vi "Calculate Flattened Indexes.vi"(4 "Q2 Q3 modifier (unreleased)":refnum<class "1D Array f32.lvclass">, 6 "Angle":refnum<class "1D Array f32.lvclass">, 7 "Image Size":sgl, 8 "error in (no error)":errorcluster, 9 "Relative X (unreleased)":refnum<class "1D Array f32.lvclass">, 10 "Relative Y (unreleased)":refnum<class "1D Array f32.lvclass">, 11 "Range In (unreleased)":refnum<class "2D Array f32.lvclass">) -> (0 "error out":errorcluster, 3 "Range Out":refnum<class "2D Array f32.lvclass">)   [LabVIEW 2020, in "G2CPU Line Profile.lvlib"]
uses:
  G2CPU Line Profile.lvlib
  <vilib>/Natan Biesmans/G2CPU GPU and CPU HPC Toolkit/G2CPU Libraries/Arrays/2DArray/f32/2D Array f32.lvclass
  C:/Program Files/National Instruments/LabVIEW 2025/vi.lib/Natan Biesmans/G2CPU GPU and CPU HPC Toolkit/G2CPU Libraries/Arrays/Array/Array Prototype.lvclass
  <vilib>/Natan Biesmans/G2CPU GPU and CPU HPC Toolkit/G2CPU Libraries/Arrays/1DArray/f32/1D Array f32.lvclass
  <vilib>/Natan Biesmans/G2CPU GPU and CPU HPC Toolkit/G2CPU Libraries/Arrays/Array/Array Prototype.lvclass/Array Prototype.ctl
  d14302c9-1abf-46cd-b8e1-cfd88139205b.vi
  3f418511-01e8-4418-a7b9-049296d044c6.vi
  6ff3651a-7429-4d59-9dc9-6d2307288a37.vi
  9237495b-07c2-4526-b901-02e97fb6c373.vi
  5aff2ad7-f89e-4eb8-8bcb-749f2898e5ad.vi
  8b20bb11-a6a9-4062-83c0-ddef68e428b2.vi
  <vilib>/Natan Biesmans/G2CPU GPU and CPU HPC Toolkit/G2CPU Libraries/Arrays/Array/G2CPU Get Array Pointer.vi
  d14302c9-1abf-46cd-b8e1-cfd88139205b.vi/6197f869-f6d4-49b3-9b2c-cc979b422c2e.vi
  d14302c9-1abf-46cd-b8e1-cfd88139205b.vi/a7e86dbb-b4c0-485c-89c5-522e60ee265c.vi
  3f418511-01e8-4418-a7b9-049296d044c6.vi/5793b77b-c002-4ebf-9075-685617c95341.vi
  3f418511-01e8-4418-a7b9-049296d044c6.vi/2ed3ef86-c00d-4d71-b84c-20267a6dfcf9.vi
  6ff3651a-7429-4d59-9dc9-6d2307288a37.vi/5793b77b-c002-4ebf-9075-685617c95341.vi
  6ff3651a-7429-4d59-9dc9-6d2307288a37.vi/2ed3ef86-c00d-4d71-b84c-20267a6dfcf9.vi
  9237495b-07c2-4526-b901-02e97fb6c373.vi/6197f869-f6d4-49b3-9b2c-cc979b422c2e.vi
  9237495b-07c2-4526-b901-02e97fb6c373.vi/a7e86dbb-b4c0-485c-89c5-522e60ee265c.vi
  5aff2ad7-f89e-4eb8-8bcb-749f2898e5ad.vi/6197f869-f6d4-49b3-9b2c-cc979b422c2e.vi
  5aff2ad7-f89e-4eb8-8bcb-749f2898e5ad.vi/a7e86dbb-b4c0-485c-89c5-522e60ee265c.vi
  8b20bb11-a6a9-4062-83c0-ddef68e428b2.vi/5793b77b-c002-4ebf-9075-685617c95341.vi
  8b20bb11-a6a9-4062-83c0-ddef68e428b2.vi/2ed3ef86-c00d-4d71-b84c-20267a6dfcf9.vi
  d14302c9-1abf-46cd-b8e1-cfd88139205b.vi/6197f869-f6d4-49b3-9b2c-cc979b422c2e.vi/3e802c67-fb96-46a3-ae13-4994a8508b4f.vi
  d14302c9-1abf-46cd-b8e1-cfd88139205b.vi/6197f869-f6d4-49b3-9b2c-cc979b422c2e.vi/5a50fc67-79e7-4972-80c2-92243cd53dd4.vi
  d14302c9-1abf-46cd-b8e1-cfd88139205b.vi/6197f869-f6d4-49b3-9b2c-cc979b422c2e.vi/1c928fc9-710a-40e7-8c4f-08a1069452ae.vi
  d14302c9-1abf-46cd-b8e1-cfd88139205b.vi/a7e86dbb-b4c0-485c-89c5-522e60ee265c.vi/730f6c57-5c0b-4ee9-b61e-75067b25222b.vi
  d14302c9-1abf-46cd-b8e1-cfd88139205b.vi/a7e86dbb-b4c0-485c-89c5-522e60ee265c.vi/096b8799-7810-404e-baca-ba9279cec4bd.vi
  d14302c9-1abf-46cd-b8e1-cfd88139205b.vi/a7e86dbb-b4c0-485c-89c5-522e60ee265c.vi/0f1a5a47-bcc5-4796-ac31-8dfcfbc0d7d1.vi
  d14302c9-1abf-46cd-b8e1-cfd88139205b.vi/a7e86dbb-b4c0-485c-89c5-522e60ee265c.vi/89f12e17-3330-4b72-ad8f-8dd636660732.vi
  3f418511-01e8-4418-a7b9-049296d044c6.vi/5793b77b-c002-4ebf-9075-685617c95341.vi/3e802c67-fb96-46a3-ae13-4994a8508b4f.vi
  3f418511-01e8-4418-a7b9-049296d044c6.vi/5793b77b-c002-4ebf-9075-685617c95341.vi/5a50fc67-79e7-4972-80c2-92243cd53dd4.vi
  3f418511-01e8-4418-a7b9-049296d044c6.vi/2ed3ef86-c00d-4d71-b84c-20267a6dfcf9.vi/730f6c57-5c0b-4ee9-b61e-75067b25222b.vi
  3f418511-01e8-4418-a7b9-049296d044c6.vi/2ed3ef86-c00d-4d71-b84c-20267a6dfcf9.vi/096b8799-7810-404e-baca-ba9279cec4bd.vi
  3f418511-01e8-4418-a7b9-049296d044c6.vi/2ed3ef86-c00d-4d71-b84c-20267a6dfcf9.vi/0f1a5a47-bcc5-4796-ac31-8dfcfbc0d7d1.vi
  3f418511-01e8-4418-a7b9-049296d044c6.vi/2ed3ef86-c00d-4d71-b84c-20267a6dfcf9.vi/89f12e17-3330-4b72-ad8f-8dd636660732.vi
  6ff3651a-7429-4d59-9dc9-6d2307288a37.vi/5793b77b-c002-4ebf-9075-685617c95341.vi/3e802c67-fb96-46a3-ae13-4994a8508b4f.vi
  6ff3651a-7429-4d59-9dc9-6d2307288a37.vi/5793b77b-c002-4ebf-9075-685617c95341.vi/5a50fc67-79e7-4972-80c2-92243cd53dd4.vi
  6ff3651a-7429-4d59-9dc9-6d2307288a37.vi/5793b77b-c002-4ebf-9075-685617c95341.vi/1c928fc9-710a-40e7-8c4f-08a1069452ae.vi
  6ff3651a-7429-4d59-9dc9-6d2307288a37.vi/2ed3ef86-c00d-4d71-b84c-20267a6dfcf9.vi/730f6c57-5c0b-4ee9-b61e-75067b25222b.vi
  6ff3651a-7429-4d59-9dc9-6d2307288a37.vi/2ed3ef86-c00d-4d71-b84c-20267a6dfcf9.vi/096b8799-7810-404e-baca-ba9279cec4bd.vi
  6ff3651a-7429-4d59-9dc9-6d2307288a37.vi/2ed3ef86-c00d-4d71-b84c-20267a6dfcf9.vi/0f1a5a47-bcc5-4796-ac31-8dfcfbc0d7d1.vi
  6ff3651a-7429-4d59-9dc9-6d2307288a37.vi/2ed3ef86-c00d-4d71-b84c-20267a6dfcf9.vi/89f12e17-3330-4b72-ad8f-8dd636660732.vi
  9237495b-07c2-4526-b901-02e97fb6c373.vi/6197f869-f6d4-49b3-9b2c-cc979b422c2e.vi/3e802c67-fb96-46a3-ae13-4994a8508b4f.vi
  9237495b-07c2-4526-b901-02e97fb6c373.vi/6197f869-f6d4-49b3-9b2c-cc979b422c2e.vi/5a50fc67-79e7-4972-80c2-92243cd53dd4.vi
  9237495b-07c2-4526-b901-02e97fb6c373.vi/a7e86dbb-b4c0-485c-89c5-522e60ee265c.vi/730f6c57-5c0b-4ee9-b61e-75067b25222b.vi
  9237495b-07c2-4526-b901-02e97fb6c373.vi/a7e86dbb-b4c0-485c-89c5-522e60ee265c.vi/096b8799-7810-404e-baca-ba9279cec4bd.vi
  9237495b-07c2-4526-b901-02e97fb6c373.vi/a7e86dbb-b4c0-485c-89c5-522e60ee265c.vi/0f1a5a47-bcc5-4796-ac31-8dfcfbc0d7d1.vi
  9237495b-07c2-4526-b901-02e97fb6c373.vi/a7e86dbb-b4c0-485c-89c5-522e60ee265c.vi/89f12e17-3330-4b72-ad8f-8dd636660732.vi
  5aff2ad7-f89e-4eb8-8bcb-749f2898e5ad.vi/6197f869-f6d4-49b3-9b2c-cc979b422c2e.vi/3e802c67-fb96-46a3-ae13-4994a8508b4f.vi
  5aff2ad7-f89e-4eb8-8bcb-749f2898e5ad.vi/6197f869-f6d4-49b3-9b2c-cc979b422c2e.vi/5a50fc67-79e7-4972-80c2-92243cd53dd4.vi
  5aff2ad7-f89e-4eb8-8bcb-749f2898e5ad.vi/a7e86dbb-b4c0-485c-89c5-522e60ee265c.vi/730f6c57-5c0b-4ee9-b61e-75067b25222b.vi
  5aff2ad7-f89e-4eb8-8bcb-749f2898e5ad.vi/a7e86dbb-b4c0-485c-89c5-522e60ee265c.vi/096b8799-7810-404e-baca-ba9279cec4bd.vi
  5aff2ad7-f89e-4eb8-8bcb-749f2898e5ad.vi/a7e86dbb-b4c0-485c-89c5-522e60ee265c.vi/0f1a5a47-bcc5-4796-ac31-8dfcfbc0d7d1.vi
  5aff2ad7-f89e-4eb8-8bcb-749f2898e5ad.vi/a7e86dbb-b4c0-485c-89c5-522e60ee265c.vi/89f12e17-3330-4b72-ad8f-8dd636660732.vi
  8b20bb11-a6a9-4062-83c0-ddef68e428b2.vi/5793b77b-c002-4ebf-9075-685617c95341.vi/3e802c67-fb96-46a3-ae13-4994a8508b4f.vi
  8b20bb11-a6a9-4062-83c0-ddef68e428b2.vi/5793b77b-c002-4ebf-9075-685617c95341.vi/5a50fc67-79e7-4972-80c2-92243cd53dd4.vi
  8b20bb11-a6a9-4062-83c0-ddef68e428b2.vi/2ed3ef86-c00d-4d71-b84c-20267a6dfcf9.vi/730f6c57-5c0b-4ee9-b61e-75067b25222b.vi
  8b20bb11-a6a9-4062-83c0-ddef68e428b2.vi/2ed3ef86-c00d-4d71-b84c-20267a6dfcf9.vi/096b8799-7810-404e-baca-ba9279cec4bd.vi
  8b20bb11-a6a9-4062-83c0-ddef68e428b2.vi/2ed3ef86-c00d-4d71-b84c-20267a6dfcf9.vi/0f1a5a47-bcc5-4796-ac31-8dfcfbc0d7d1.vi
  8b20bb11-a6a9-4062-83c0-ddef68e428b2.vi/2ed3ef86-c00d-4d71-b84c-20267a6dfcf9.vi/89f12e17-3330-4b72-ad8f-8dd636660732.vi
  <vilib>/Natan Biesmans/G2CPU GPU and CPU HPC Toolkit/ArrayFire Driver/VIs/Run as Multi Device.vi
  d14302c9-1abf-46cd-b8e1-cfd88139205b.vi/6197f869-f6d4-49b3-9b2c-cc979b422c2e.vi/3e802c67-fb96-46a3-ae13-4994a8508b4f.vi/1b7cf390-2ae0-48f3-9bce-03c57eed6ee8.vi
  6ff3651a-7429-4d59-9dc9-6d2307288a37.vi/5793b77b-c002-4ebf-9075-685617c95341.vi/3e802c67-fb96-46a3-ae13-4994a8508b4f.vi/1b7cf390-2ae0-48f3-9bce-03c57eed6ee8.vi
  9237495b-07c2-4526-b901-02e97fb6c373.vi/a7e86dbb-b4c0-485c-89c5-522e60ee265c.vi/730f6c57-5c0b-4ee9-b61e-75067b25222b.vi/0070e0fe-4ad7-4a3e-8965-d64becb7e5f0.vi
  5aff2ad7-f89e-4eb8-8bcb-749f2898e5ad.vi/a7e86dbb-b4c0-485c-89c5-522e60ee265c.vi/730f6c57-5c0b-4ee9-b61e-75067b25222b.vi/0070e0fe-4ad7-4a3e-8965-d64becb7e5f0.vi
  <vilib>/Natan Biesmans/G2CPU GPU and CPU HPC Toolkit/ArrayFire Driver/subvi/Error Converter (ErrCode or Status).vi
  <vilib>/Natan Biesmans/G2CPU GPU and CPU HPC Toolkit/G2CPU Libraries/Arrays/Array/G2CPU Set Array Pointer.vi
  <vilib>/Natan Biesmans/G2CPU GPU and CPU HPC Toolkit/G2CPU Libraries/Arrays/SubVI/is 1D.vi
  <vilib>/Natan Biesmans/G2CPU GPU and CPU HPC Toolkit/ArrayFire Driver/VIs/mul.vi
  <vilib>/Natan Biesmans/G2CPU GPU and CPU HPC Toolkit/G2CPU Libraries/Arrays/Array/G2CPU Release Array.vi
  <vilib>/Natan Biesmans/G2CPU GPU and CPU HPC Toolkit/ArrayFire Driver/VIs/add.vi
  <vilib>/Natan Biesmans/G2CPU GPU and CPU HPC Toolkit/G2CPU Libraries/Arrays/SubVI/is 2D.vi
  <vilib>/Natan Biesmans/G2CPU GPU and CPU HPC Toolkit/G2CPU Libraries/Arrays/DataTypes/f32/f32.lvclass
  <vilib>/Natan Biesmans/G2CPU GPU and CPU HPC Toolkit/G2CPU Libraries/Arrays/1DArray/1D Array Prototype.lvclass
  <vilib>/Natan Biesmans/G2CPU GPU and CPU HPC Toolkit/G2CPU Libraries/Arrays/Array/Array Prototype.lvclass
  <vilib>/Natan Biesmans/G2CPU GPU and CPU HPC Toolkit/G2CPU Libraries/Arrays/2DArray/2D Array Prototype.lvclass
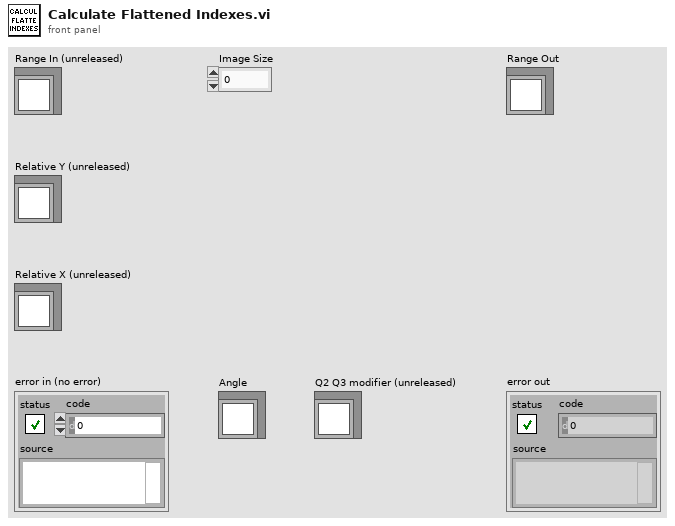
[diagram p1: front panel]
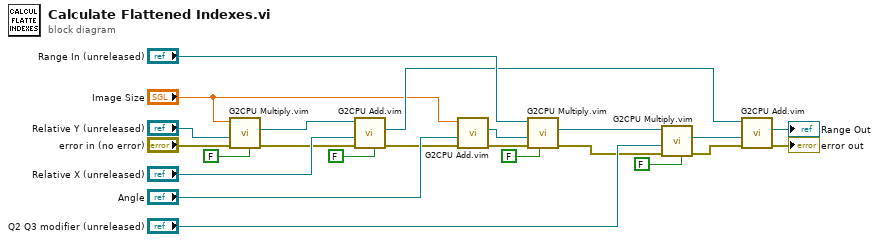
[diagram p0: block diagram]
diagram:
  n1 = call "G2CPU Multiply.vim"("Auto Release rhs"=FALSE, "error in (no error)"="error in (no error)", "Array rhs"="Relative Y (unreleased)", "Array lhs"="Image Size") -> ("error out"=w8:errorcluster, "Array Result"=w19:refnum<class "1D Array f32.lvclass">)  [unwired: 6 in]
  n2 = call "G2CPU Add.vim"("Auto Release rhs (Enabled)"=FALSE, "error in (no error)"=w8, "Array rhs"="Relative X (unreleased)", "Array lhs"=w19) -> ("error out"=w7:errorcluster, "Array Result"=w18:refnum<class "1D Array f32.lvclass">)  [unwired: 6 in]
  n3 = call "G2CPU Add.vim"("error in (no error)"=w7, "Array rhs"="Angle", "Array lhs"="Image Size") -> ("error out"=w6:errorcluster, "Array Result"=w17:refnum<class "1D Array f32.lvclass">)  [unwired: 7 in]
  n4 = call "G2CPU Multiply.vim"("Auto Release lhs"=FALSE, "error in (no error)"=w6, "Array rhs"=w17, "Array lhs"="Range In (unreleased)") -> ("error out"=w5:errorcluster, "Array Result"=w12:refnum<class "2D Array f32.lvclass">)  [unwired: 6 in]
  n5 = call "G2CPU Multiply.vim"("Auto Release rhs"=FALSE, "error in (no error)"=w5, "Array rhs"="Q2 Q3 modifier (unreleased)", "Array lhs"=w12) -> ("error out"=w4:errorcluster, "Array Result"=w11:refnum<class "2D Array f32.lvclass">)  [unwired: 6 in]
  n6 = call "G2CPU Add.vim"("error in (no error)"=w4, "Array rhs"=w11, "Array lhs"=w18) -> ("error out"=→"error out":errorcluster, "Array Result"=→"Range Out":refnum<class "2D Array f32.lvclass">)  [unwired: 7 in]
